vi "Main.vi"() -> ()   [LabVIEW 2024]
doc: "This small application is only a proof of concept. When we have parameters or user data inside an application that could be modified (by the user) at run time, it is important that those changes are 'memorized' when the application is shut down. The next time the application is started it should keep the last configuration made. This is what this application does.\n\nEvery time the user changes the FP data, the changes are saved in the .ini file. If the user closes the application, the FP data is already saved in the .ini configuration file. The next time it is turned on, the data will be loaded again.\n\nIf the user modifies any tag or sector name, or any key name (or its value) in the configuration file (and saves these changes) at run time, the Update button updates this information in the FP of the application, it is the data of the gray fields. This may not be useful in a real application."
uses:
  controls/UI Data.ctl
  controls/ring data.ctl
  support/Message Queue/Enqueue Message (Array).vi
  support/Message Queue/Enqueue Message (Single).vi
  dependencies/read-write config ini string data.vi
  <vilib>/Utility/config.llb/Read Key (String).vi
  <vilib>/Utility/config.llb/Write Key (String).vi
  <vilib>/Utility/error.llb/Error Cluster From Error Code.vi
  <vilib>/ErrorRing/Error Ring.xnode
  support/Message Queue/Message Queue.lvlib
  support/User Event - Stop/User Event - Stop.lvlib
  dependencies/read-write config ini.lvlib
  <vilib>/Utility/config.llb/NI_LVConfig.lvlib
panel:
  in  "Capacity":u16(ring) items=["9k", "12k", "18k", "24k"]
  in  "Type":u16(ring) items=["AB ROS", "INVERTER AG", "INVERTER SAMSUNG"]
  in  "Chassis":u16(ring) items=["MIDEA", "TCL"]
  in  "Sequence":u16(ring) items=["LOW", "LOW,MID", "LOW,HIGH", "LOW,TURBO", "LOW,MID,HIGH", "LOW,MID,TURBO", "LOW,HIGH,TURBO", "LOW,MID,HIGH,TURBO"]
  out "Display value":string
  in  "Exit":bool
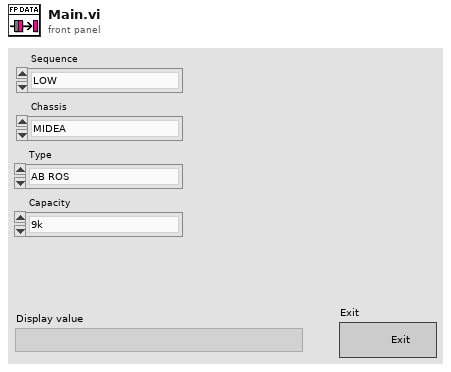
[diagram p1: front panel]
types:
  T1 = typedef "UI Data.ctl" = cluster{"Data Display Ref":refnum<vi>, "Exit Button Ref":refnum<vi>, "Ring Ref":refnum<vi>[], "types by chassis":T2, "ring opts":T2, "user ring data":T2, "actual chassis":string, "opt new type":cluster{"type":string, "key names":string[], "key values":string[]}}
  T2 = typedef "ring data.ctl" = cluster{"sectors":string[][], "key names":string[], "values":string[]}
  T3 = typedef "Message Queue.lvlib/All Message Queues.ctl" = cluster{"UI":refnum<queue>}
  T4 = cluster{"type":string, "key names":string[], "key values":string[]}
  T5 = typedef "NI_LVConfig.lvlib/Config Data RefNum.ctl" = refnum<k1>
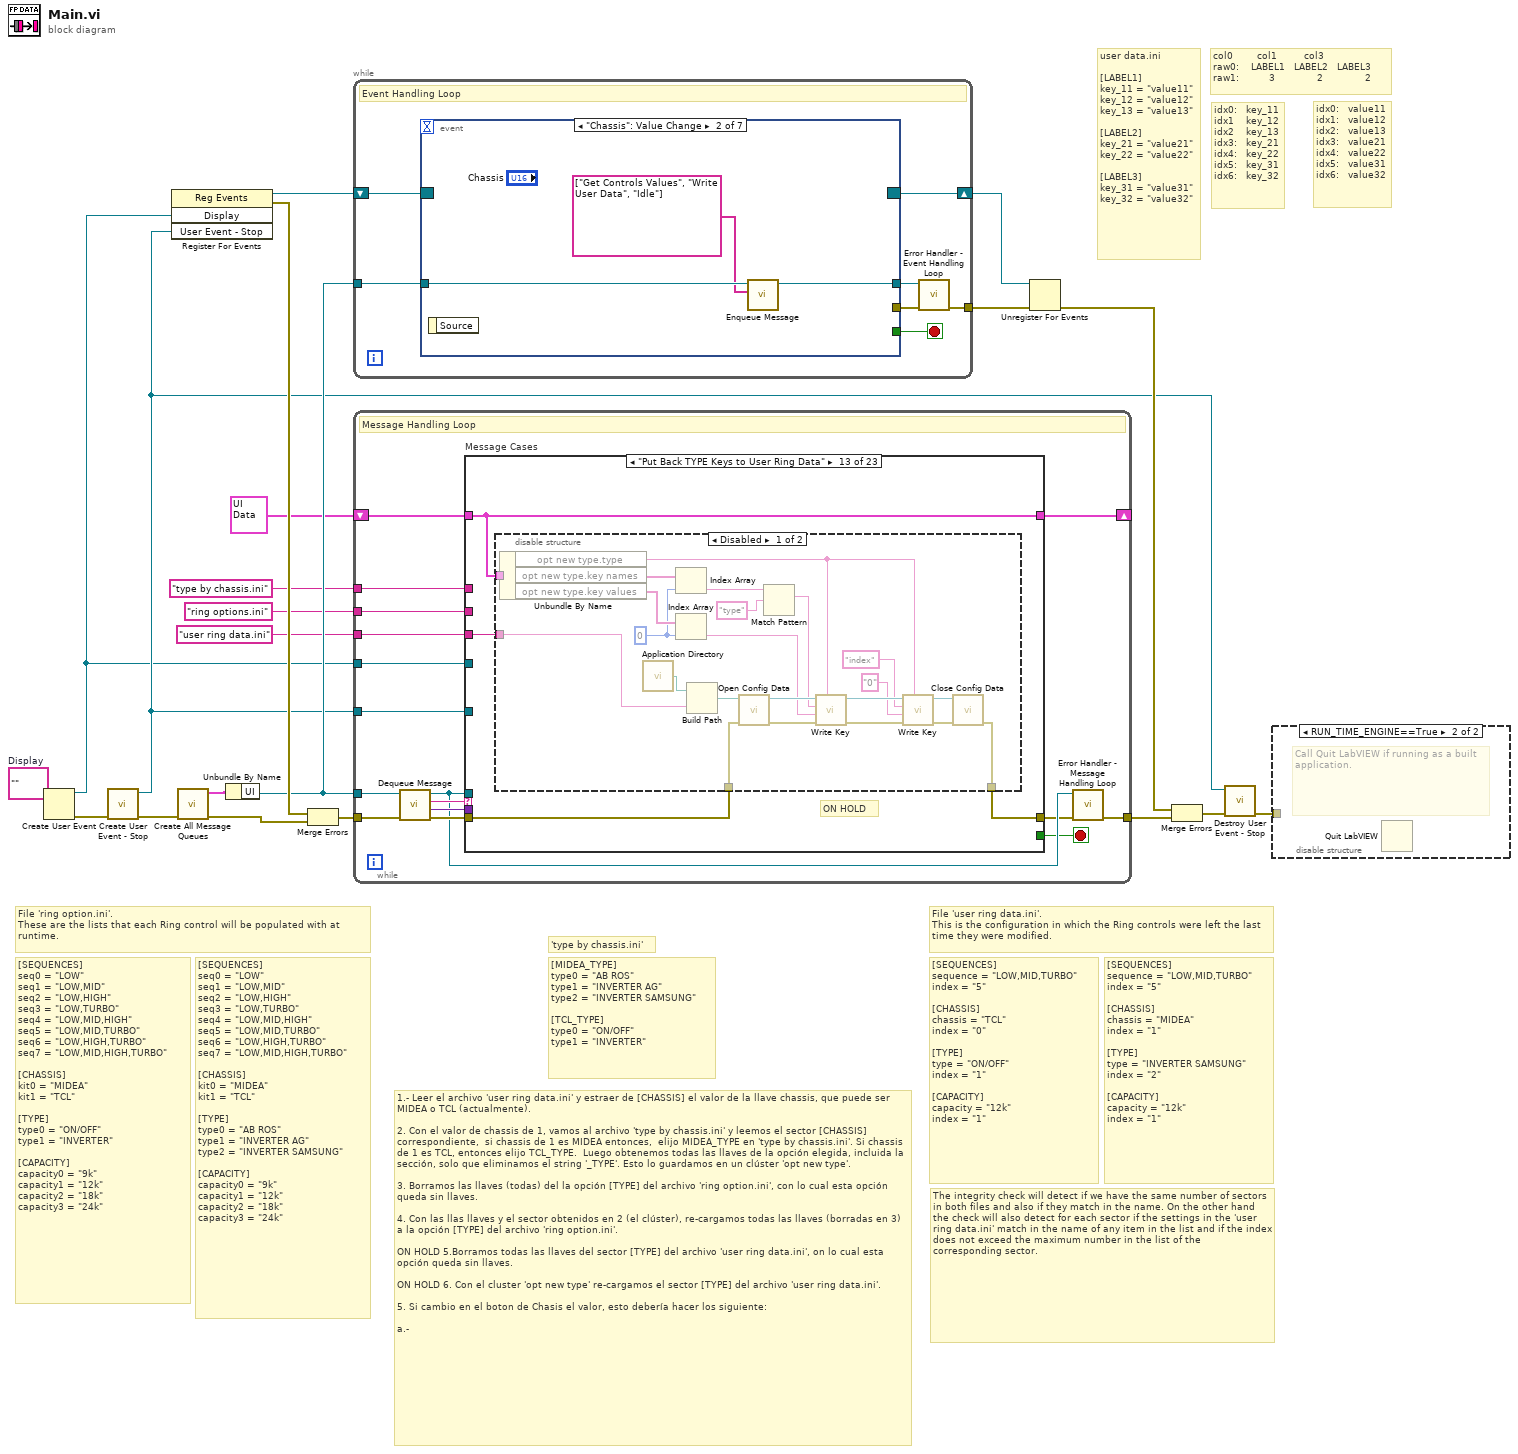
[diagram p0: block diagram]
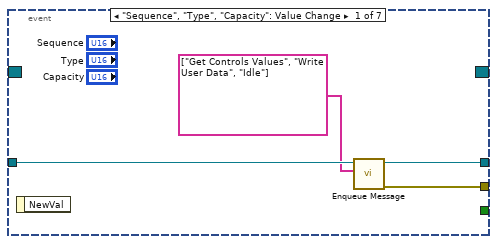
[diagram p3: hidden frame]
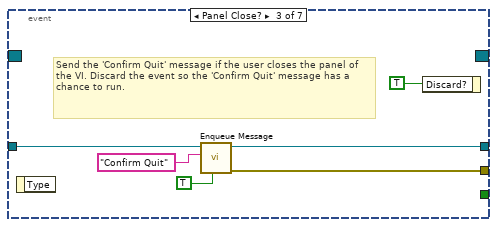
[diagram p4: hidden frame]
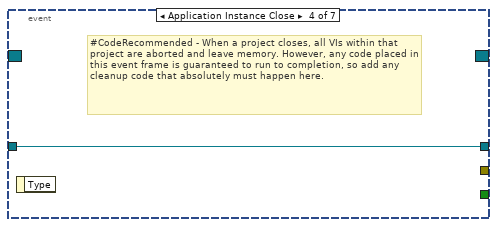
[diagram p5: hidden frame]
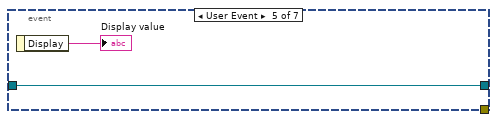
[diagram p6: hidden frame]
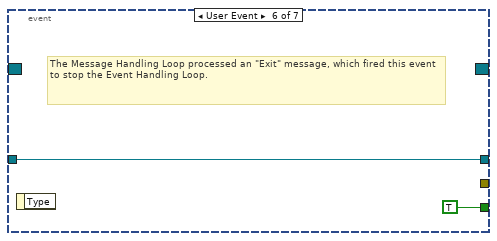
[diagram p7: hidden frame]
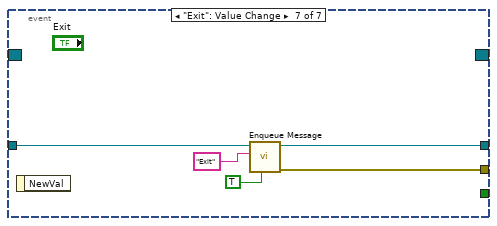
[diagram p8: hidden frame]
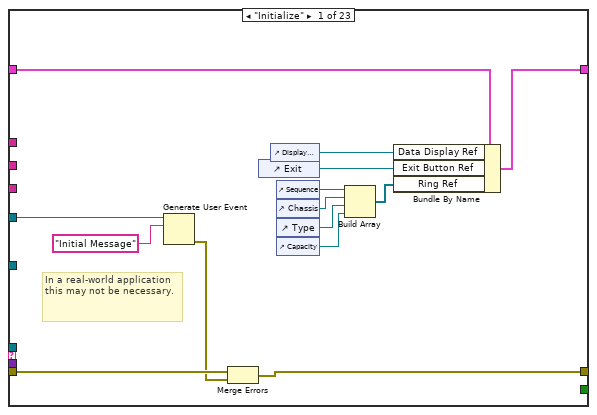
[diagram p9: hidden frame]
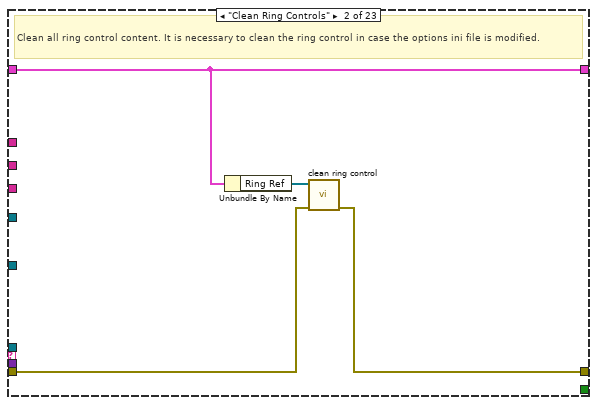
[diagram p10: hidden frame]
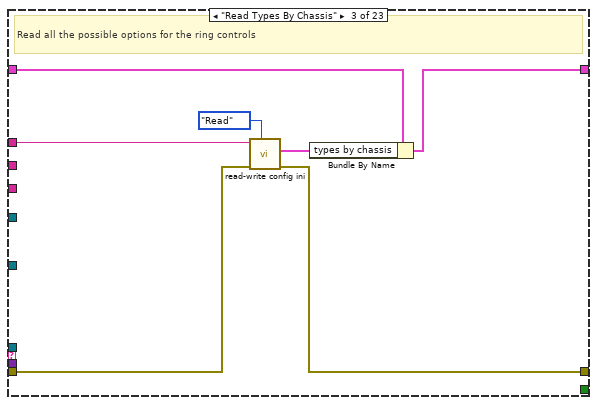
[diagram p11: hidden frame]
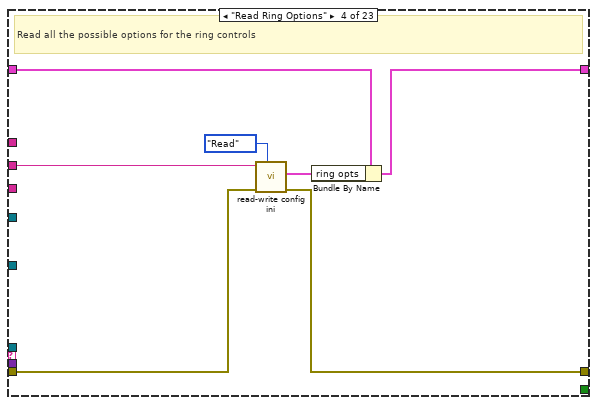
[diagram p12: hidden frame]
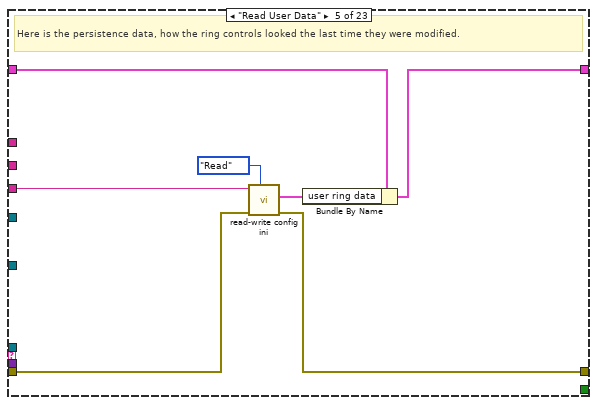
[diagram p13: hidden frame]
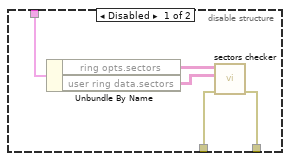
[diagram p15: hidden frame]
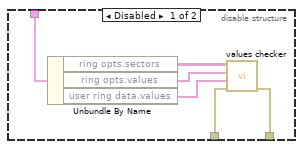
[diagram p17: hidden frame]
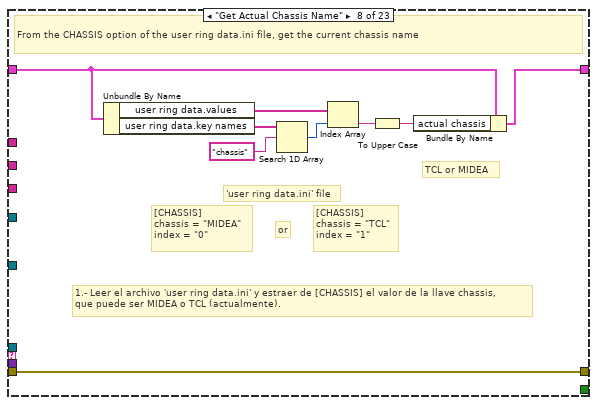
[diagram p18: hidden frame]
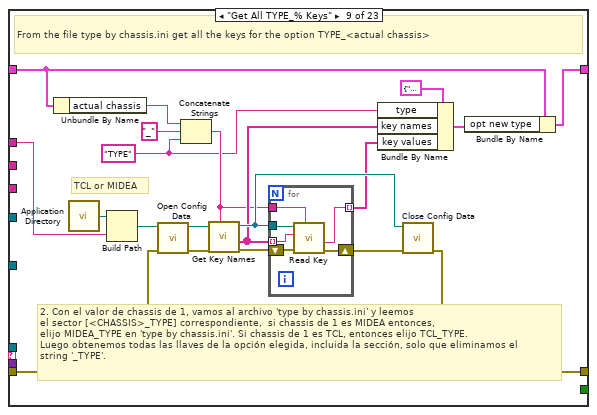
[diagram p19: hidden frame]
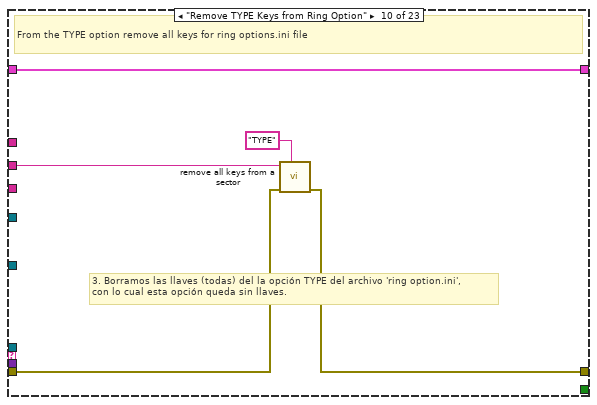
[diagram p20: hidden frame]
diagram:
  w6 = ""  # Display
  # "1.- Leer el archivo 'user ring data.ini' y estraer de [CHASSIS] el valor de la llave chassis, que puede ser MIDEA o TCL (actualmente).\n\n2. Con el valor de chassis de 1, vamos al archivo 'type by chassis.ini' y leemos el sector [CHASSIS] correspondiente,  si chassis de 1 es MIDEA entonces,  elijo MIDEA_TYPE en 'type by chassis.ini'. Si chassis de 1 es TCL, entonces elijo TCL_TYPE.  Luego obtenemos todas las llaves de la opción elegida, incluida la sección, solo que eliminamos el string '_TYPE'. Esto lo guardamos en un clúster 'opt new type'.\n\n3. Borramos las llaves (todas) del la opción [TYPE] del archivo 'ring option.ini', con lo cual esta opción queda sin llaves.\n\n4. Con las llas llaves y el sector obtenidos en 2 (el clúster), re-cargamos todas las llaves (borradas en 3) a la opción [TYPE] del archivo 'ring option.ini'.\n\nON HOLD 5.Borramos todas las llaves del sector [TYPE] del archivo 'user ring data.ini', on lo cual esta opción queda sin llaves.\n\nON HOLD 6. Con el cluster 'opt new type' re-cargamos el sector [TYPE] del archivo 'user ring data.ini'.\n\n5. Si cambio en el boton de Chasis el valor, esto debería hacer los siguiente:\n\na.-"
  # "[SEQUENCES]\nsequence = \"LOW,MID,TURBO\"\nindex = \"5\"\n\n[CHASSIS]\nchassis = \"MIDEA\"\nindex = \"1\"\n\n[TYPE]\ntype = \"INVERTER SAMSUNG\"\nindex = \"2\"\n\n[CAPACITY]\ncapacity = \"12k\"\nindex = \"1\""
  # "[SEQUENCES]\nseq0 = \"LOW\"\nseq1 = \"LOW,MID\"\nseq2 = \"LOW,HIGH\"\nseq3 = \"LOW,TURBO\"\nseq4 = \"LOW,MID,HIGH\"\nseq5 = \"LOW,MID,TURBO\"\nseq6 = \"LOW,HIGH,TURBO\"\nseq7 = \"LOW,MID,HIGH,TURBO\"\n\n[CHASSIS]\nkit0 = \"MIDEA\"\nkit1 = \"TCL\"\n\n[TYPE]\ntype0 = \"ON/OFF\"\ntype1 = \"INVERTER\"\n\n[CAPACITY]\ncapacity0 = \"9k\"\ncapacity1 = \"12k\"\ncapacity2 = \"18k\"\ncapacity3 = \"24k\""
  # "[MIDEA_TYPE]\ntype0 = \"AB ROS\"\ntype1 = \"INVERTER AG\"\ntype2 = \"INVERTER SAMSUNG\"\n\n[TCL_TYPE]\ntype0 = \"ON/OFF\"\ntype1 = \"INVERTER\""
  # "'type by chassis.ini'"
  # "The integrity check will detect if we have the same number of sectors in both files and also if they match in the name. On the other hand the check will also detect for each sector if the settings in the 'user ring data.ini' match in the name of any item in the list and if the index does not exceed the maximum number in the list of the corresponding sector."
  # "File 'user ring data.ini'.\nThis is the configuration in which the Ring controls were left the last time they were modified."
  # "[SEQUENCES]\nsequence = \"LOW,MID,TURBO\"\nindex = \"5\"\n\n[CHASSIS]\nchassis = \"TCL\"\nindex = \"0\"\n\n[TYPE]\ntype = \"ON/OFF\"\nindex = \"1\"\n\n[CAPACITY]\ncapacity = \"12k\"\nindex = \"1\""
  # "File 'ring option.ini'.\nThese are the lists that each Ring control will be populated with at runtime."
  # "[SEQUENCES]\nseq0 = \"LOW\"\nseq1 = \"LOW,MID\"\nseq2 = \"LOW,HIGH\"\nseq3 = \"LOW,TURBO\"\nseq4 = \"LOW,MID,HIGH\"\nseq5 = \"LOW,MID,TURBO\"\nseq6 = \"LOW,HIGH,TURBO\"\nseq7 = \"LOW,MID,HIGH,TURBO\"\n\n[CHASSIS]\nkit0 = \"MIDEA\"\nkit1 = \"TCL\"\n\n[TYPE]\ntype0 = \"AB ROS\"\ntype1 = \"INVERTER AG\"\ntype2 = \"INVERTER SAMSUNG\"\n\n[CAPACITY]\ncapacity0 = \"9k\"\ncapacity1 = \"12k\"\ncapacity2 = \"18k\"\ncapacity3 = \"24k\""
  # "user data.ini\n\n[LABEL1]\nkey_11 = \"value11\"\nkey_12 = \"value12\"\nkey_13 = \"value13\"\n\n[LABEL2]\nkey_21 = \"value21\"\nkey_22 = \"value22\"\n\n[LABEL3]\nkey_31 = \"value31\"\nkey_32 = \"value32\""
  # "idx0:   value11\nidx1:   value12\nidx2:   value13\nidx3:   value21\nidx4:   value22\nidx5:   value31\nidx6:   value32"
  # "idx0:   key_11\nidx1    key_12\nidx2    key_13\nidx3:   key_21\nidx4:   key_22\nidx5:   key_31\nidx6:   key_32"
  # "col0        col1         col3   \nraw0:    LABEL1   LABEL2   LABEL3\nraw1:          3              2              2"
  n1 = Create User Event(user event datatype=w6) -> (user event=w4:refnum<user-event>, error out=w7:errorcluster)  [unwired: 1 in]
  n2 = call "Create User Event - Stop.vi"("error in (no error)"=w7) -> ("error out"=w16:errorcluster, "User Event - Stop"=w5:refnum<user-event>)  [unwired: 9 in]
  n3 = register-events(w4, w5) -> (reference out=w9:refnum<event-registration>, error out=w21:errorcluster)  [unwired: 2 in]
  n4 = call "Create All Message Queues.vi"("error in (no error)"=w16) -> ("error out"=w20:errorcluster, "Message Queues out"=w19:T3)  [unwired: 9 in]
  n5 = Unbundle By Name(w19) -> ("UI"=w17:refnum<queue>)
  n6 = Merge Errors(w21, w20) -> (w8:errorcluster)
  n7 = while {
    tunnel: w17 -> [w28]
    shift-right: [w26] -> w13
    shift-left: w9 -> [w27]
    tunnel: [w22] -> w10
    stop <- w24 stop-if-true
    # "Event Handling Loop"
    n8 = event shown="[1] \"Chassis\": Value Change" {
      selector: w27 -> [_ _ _ _ _ _ _]
      dyn-events: [_ _ _ _ _ _ _] -> w26
      timeout: _ -> [_ _ _ _ _ _ _]
      tunnel: [_ _ _ _ _ TRUE ("Discard?") _] -> w24
      tunnel: w28 -> [w32 w35 w40 w42 w44 w46 w51]
      tunnel: [w30 _ w39 _ _ _ w50] -> w25
      tunnel: [w31 w34 w38 w42 w44 w46 w49] -> w23
      event "Sequence", "Type", "Capacity": Value Change {
        n9 = event-data() -> ()  [unwired: 1 in, 1 out]
        n10 = call-poly "Enqueue Message.vi"("Message Array"=string[] ["Get Controls Values", "Write User Data", "Idle"], "Message Queue"=w32) -> ("error out"=w30:errorcluster, "dup Message Queue"=w31:refnum<queue>)  [unwired: 8 in]
      }
      event "Chassis": Value Change {
        n11 = event-data() -> ()  [unwired: 1 in, 1 out]
        n12 = call-poly "Enqueue Message.vi"("Message Array"=string[] ["Get Controls Values", "Write User Data", "Idle"], "Message Queue"=w35) -> ("dup Message Queue"=w34:refnum<queue>)  [unwired: 8 in, 1 out]
      }
      event Panel Close? {
        # "Send the 'Confirm Quit' message if the user closes the panel of the VI. Discard the event so the 'Confirm Quit' message has a chance to run."
        n13 = event-data() -> ()  [unwired: 1 in, 1 out]
        n14 = call-poly "Enqueue Message.vi"("Priority Message? (F)"=TRUE, "Message"="Confirm Quit", "Message Queue"=w40) -> ("error out"=w39:errorcluster, "dup Message Queue"=w38:refnum<queue>)  [unwired: 7 in]
        n15 = event-data("Discard?"=TRUE) -> ()  [unwired: 1 in, 1 out]
      }
      event Application Instance Close {
        # "#CodeRecommended - When a project closes, all VIs within that project are aborted and leave memory. However, any code placed in this event frame is guaranteed to run to completion, so add any cleanup code that absolutely must happen here."
        n16 = event-data() -> ()  [unwired: 1 in, 1 out]
      }
      event User Event {
        n17 = event-data() -> ("Display"=→"Display value":string)  [unwired: 1 in]
      }
      event User Event {
        # "The Message Handling Loop processed an \"Exit\" message, which fired this event to stop the Event Handling Loop."
        n18 = event-data() -> ()  [unwired: 1 in, 1 out]
      }
      event "Exit": Value Change {
        n19 = event-data() -> ()  [unwired: 1 in, 1 out]
        n20 = call-poly "Enqueue Message.vi"("Priority Message? (F)"=TRUE, "Message"="Exit", "Message Queue"=w51) -> ("error out"=w50:errorcluster, "dup Message Queue"=w49:refnum<queue>)  [unwired: 7 in]
      }
    }
    n21 = call "Error Handler - Event Handling Loop.vi"("error in (no error)"=w25, "Message Queue"=w23) -> ("dup error in"=w22:errorcluster)  [unwired: 8 in, 1 out]
  }
  n22 = while {
    tunnel: w17 -> [w61]
    shift-right: [w56] -> _
    shift-left: T1 {"Data Display Ref"=refnum, "Exit Button Ref"=refnum, "Ring Ref"=[], "types by chassis"={"sectors"=[], "key names"=[], "values"=[]}, "ring opts"={"sectors"=[], "key names"=[], "values"=[]}, "user ring data"={"sectors"=[], "key names"=[], "values"=[]}, "actual chassis"="", "opt new type"={"type"="", "key names"=[], "key values"=[]}} ("Data Cluster") -> [w67]
    tunnel: w5 -> [w66]
    tunnel: w8 -> [w65]
    tunnel: [w59] -> w18
    tunnel: w4 -> [w57]
    tunnel: "user ring data.ini" -> [w55]
    tunnel: "ring options.ini" -> [w53]
    tunnel: "type by chassis.ini" -> [w52]
    stop <- w54 stop-if-true
    # "Message Handling Loop"
    n23 = call "Dequeue Message.vi"("error in (no error)"=w65, "Message Queue"=w61) -> ("error out"=w64:errorcluster, "Message Data"=w62:variant, "Message"=w63:string, "dup Message Queue"=w60:refnum<queue>)  [unwired: 6 in]
    n24 = case "Message Cases" shown="\"Put Back TYPE Keys to User Ring Data\"" w63 {
      selector: w63 -> [_ _ _ _ _ _ _ _ _ _ _ _ _ _ _ _ _ _ _ _ _ _ w281]
      tunnel: w60 -> [_ _ _ _ _ _ _ _ _ _ _ _ _ _ _ _ _ _ _ w259 _ w280 _]
      tunnel: w64 -> [w77 w83 w91 w97 w102 w108 w116 w132 w144 w162 w172 w183 w192 w220 w226 w232 w234 w244 w256 w263 w266 w273 _]
      tunnel: [w74 w82 w90 w96 w101 w107 w115 w132 w143 w161 w164 w182 w191 w219 w225 w231 w235 w248 w250 w261 w264 w276 w282] -> w58
      tunnel: w67 -> [w81 w85 w89 w95 w106 w109 w117 w127 w139 w163 w171 w185 w193 w218 w224 w230 w240 w249 w255 w262 w265 w279 w283]
      tunnel: [w80 w85 w87 w93 w105 w109 w117 w126 w137 w163 w171 w185 w193 w218 w224 w229 w240 w249 w255 w262 w265 w279 w283] -> w56
      tunnel: [_ _ _ _ _ _ _ _ _ _ _ _ _ _ _ _ _ _ _ _ _ TRUE _] -> w54
      tunnel: w62 -> [_ _ _ _ _ _ _ _ _ _ _ _ _ _ _ _ _ w245 w254 _ _ w270 _]
      tunnel: w66 -> [_ _ _ _ _ _ _ _ _ _ _ _ _ _ _ _ _ _ _ _ _ w275 _]
      tunnel: w57 -> [w76 _ _ _ _ _ _ _ _ _ _ _ _ _ _ _ _ w247 _ _ _ w268 _]
      tunnel: w55 -> [_ _ _ _ w104 _ _ _ _ _ _ w184 w190 _ _ _ w239 _ _ _ _ _ _]
      tunnel: w53 -> [_ _ _ w99 _ _ _ _ _ w159 w173 _ _ _ _ _ _ _ _ _ _ _ _]
      tunnel: w52 -> [_ _ w86 _ _ _ _ _ w149 _ _ _ _ _ _ _ _ _ _ _ _ _ _]
      frame "Initialize" {
        # "In a real-world application this may not be necessary."
        n25 = Generate User Event(user event=w76, event data cluster="Initial Message" ("Initial Message")) -> (error out=w73:errorcluster)  [unwired: 2 in, 1 out]
        n26 = Merge Errors(w77, w73) -> (w74:errorcluster)
        n27 = control-ref of="Exit"() -> (w78:refnum<vi>)
        n28 = control-ref of="Display value"() -> (w79:refnum<vi>)
        n29 = control-ref of="Sequence"() -> (w72:refnum<vi>)
        n30 = control-ref of="Chassis"() -> (w71:refnum<vi>)
        n31 = control-ref of="Type"() -> (w70:refnum<vi>)
        n32 = control-ref of="Capacity"() -> (w68:refnum<vi>)
        n33 = Build Array(w72, w71, w70, w68) -> (w69:refnum<vi>[])
        n34 = Bundle By Name(cluster=w81, "Data Display Ref"=w79, "Exit Button Ref"=w78, "Ring Ref"=w69) -> (w80:T1)
      }
      frame "Clean Ring Controls" {
        # "Clean all ring control content. It is necessary to clean the ring control in case the options ini file is modified."
        n35 = Unbundle By Name(w85) -> ("Ring Ref"=w84:refnum<vi>[])
        n36 = call "clean ring control.vi"("error in (no error)"=w83, "Ring Ref"=w84) -> ("error out"=w82:errorcluster)  [unwired: 9 in]
      }
      frame "Read Types By Chassis" {
        # "Read all the possible options for the ring controls"
        n37 = call-poly "read-write config ini.vi"("Function"=enum16{"Read", "Write"}."Read", "error in (no error)"=w91, "file name"=w86) -> ("error out"=w90:errorcluster, "user data out"=w88:T2)  [unwired: 7 in]
        n38 = Bundle By Name(cluster=w89, "types by chassis"=w88) -> (w87:T1)
      }
      frame "Read Ring Options" {
        # "Read all the possible options for the ring controls"
        n39 = call-poly "read-write config ini.vi"("Function"=enum16{"Read", "Write"}."Read", "error in (no error)"=w97, "file name"=w99) -> ("error out"=w96:errorcluster, "user data out"=w94:T2)  [unwired: 7 in]
        n40 = Bundle By Name(cluster=w95, "ring opts"=w94) -> (w93:T1)
      }
      frame "Read User Data" {
        # "Here is the persistence data, how the ring controls looked the last time they were modified."
        n41 = call-poly "read-write config ini.vi"("Function"=enum16{"Read", "Write"}."Read", "error in (no error)"=w102, "file name"=w104) -> ("error out"=w101:errorcluster, "user data out"=w100:T2)  [unwired: 7 in]
        n42 = Bundle By Name(cluster=w106, "user ring data"=w100) -> (w105:T1)
      }
      frame "Check for Sectors" {
        # "Verifying configuration files integrity"
        n43 = disable-structure shown="Enabled" {
          disable-tunnel: w109 -> [w112 _]
          disable-tunnel: w108 -> [w111 _]
          disable-tunnel: [w110 _] -> w107
          frame Disabled {
            n44 = Unbundle By Name(w112) -> ("ring opts.sectors"=w114:string[][], "user ring data.sectors"=w113:string[][])
            n45 = call "sectors checker.vi"("error in (no error)"=w111, "array2"=w113, "array1"=w114) -> ("error out"=w110:errorcluster)  [unwired: 8 in]
          }
          frame Enabled {
          }
        }
      }
      frame "Check For Values" {
        # "Verifying configuration files integrity"
        n46 = disable-structure shown="Enabled" {
          disable-tunnel: w117 -> [w120 _]
          disable-tunnel: w116 -> [w119 _]
          disable-tunnel: [w118 _] -> w115
          frame Disabled {
            n47 = Unbundle By Name(w120) -> ("ring opts.sectors"=w123:string[][], "ring opts.values"=w122:string[], "user ring data.values"=w121:string[])
            n48 = call "values checker.vi"("error in (no error)"=w119, "values"=w121, "values 2"=w122, "sectors"=w123) -> ("error out"=w118:errorcluster)  [unwired: 7 in]
          }
          frame Enabled {
          }
        }
      }
      frame "Get Actual Chassis Name" {
        # "1.- Leer el archivo 'user ring data.ini' y estraer de [CHASSIS] el valor de la llave chassis, \nque puede ser MIDEA o TCL (actualmente)."
        # "TCL or MIDEA"
        # "'user ring data.ini' file"
        # "or"
        # "[CHASSIS]\nchassis = \"MIDEA\"\nindex = \"0\""
        # "[CHASSIS]\nchassis = \"TCL\"\nindex = \"1\""
        # "From the CHASSIS option of the user ring data.ini file, get the current chassis name"
        n49 = Unbundle By Name(w127) -> ("user ring data.values"=w129:string[], "user ring data.key names"=w131:string[])
        n50 = Search 1D Array(1D array=w131, element="chassis") -> (index of element=w128:i32)  [unwired: 1 in]
        n51 = Index Array(array=w129, index=w128) -> (element=w125:string)
        n52 = To Upper Case(1:w125) -> (0:w124:string)
        n53 = Bundle By Name(cluster=w127, "actual chassis"=w124) -> (w126:T1)
      }
      frame "Get All TYPE_% Keys" {
        w133 = "TYPE"
        # "2. Con el valor de chassis de 1, vamos al archivo 'type by chassis.ini' y leemos\nel sector [<CHASSIS>_TYPE] correspondiente,  si chassis de 1 es MIDEA entonces,  \nelijo MIDEA_TYPE en 'type by chassis.ini'. Si chassis de 1 es TCL, entonces elijo TCL_TYPE. \nLuego obtenemos todas las llaves de la opción elegida, incluida la sección, solo que eliminamos el \nstring '_TYPE'."
        # "TCL or MIDEA"
        # "From the file type by chassis.ini get all the keys for the option TYPE_<actual chassis>"
        n54 = Unbundle By Name(w139) -> ("actual chassis"=w134:string)
        n55 = call <vilib>:"Application Directory.vi"() -> ("Application Directory"=w151:path)
        n56 = Build Path(base path=w151, name or relative path=w149) -> (appended path=w150:path)
        n57 = call <vilib>:"Open Config Data.vi"("error in (no error)"=w144, "configuration file path"=w150) -> ("error out"=w148:errorcluster, "refnum"=w147:T5)  [unwired: 7 in, 1 out]
        n58 = Concatenate Strings(w134, "_", w133) -> (w136:string)
        n59 = call <vilib>:"Get Key Names.vi"("section"=w136, "error in (no error)"=w148, "refnum"=w147) -> ("error out"=w146:errorcluster, "key names"=w141:string[], "refnum out"=w152:T5)  [unwired: 5 in, 1 out]
        n60 = for {
          tunnel: w141 -> [w157] mode=indexing
          tunnel: w152 -> [w158]
          tunnel: w136 -> [w156]
          tunnel: [w155] -> w140 mode=indexing
          shift-right: [w153] -> w145
          shift-left: w146 -> [w154]
          n61 = call-poly <vilib>:"Read Key.vi"("section"=w156, "error in (no error)"=w154, "key"=w157, "refnum"=w158) -> ("error out"=w153:errorcluster, "value"=w155:string)  [unwired: 4 in, 2 out]
        }
        n62 = Bundle By Name(cluster=T4 {"type"="", "key names"=[], "key values"=[]}, "type"=w133, "key names"=w141, "key values"=w140) -> (w138:T4)
        n63 = call <vilib>:"Close Config Data.vi"("error in (no error)"=w145, "refnum"=w152) -> ("error out"=w143:errorcluster)  [unwired: 8 in, 1 out]
        n64 = Bundle By Name(cluster=w139, "opt new type"=w138) -> (w137:T1)
      }
      frame "Remove TYPE Keys from Ring Option" {
        # "3. Borramos las llaves (todas) del la opción TYPE del archivo 'ring option.ini', \ncon lo cual esta opción queda sin llaves."
        # "From the TYPE option remove all keys for ring options.ini file"
        n65 = call "remove all keys from a sector.vi"("sector"="TYPE", "error in (no error)"=w162, "file name"=w159) -> ("error out"=w161:errorcluster)  [unwired: 8 in]
      }
      frame "Put Back TYPE Keys to Ring Option" {
        # "4. Con las llas llaves y el sector obtenidos en 2, re-cargar todas las llaves (borradas en 3)\na la opción TYPE del archivo 'ring option.ini'."
        n66 = Unbundle By Name(w171) -> ("opt new type.type"=w169:string, "opt new type.key names"=w167:string[], "opt new type.key values"=w168:string[])
        n67 = call <vilib>:"Application Directory.vi"() -> ("Application Directory"=w174:path)
        n68 = Build Path(base path=w174, name or relative path=w173) -> (appended path=w175:path)
        n69 = call <vilib>:"Open Config Data.vi"("error in (no error)"=w172, "configuration file path"=w175) -> ("error out"=w170:errorcluster, "refnum"=w165:T5)  [unwired: 7 in, 1 out]
        n70 = for {
          tunnel: w165 -> [w180]
          tunnel: w169 -> [w179]
          shift-right: [w178] -> w166
          shift-left: w170 -> [w181]
          tunnel: w168 -> [w177] mode=indexing
          tunnel: w167 -> [w176] mode=indexing
          n71 = call-poly <vilib>:"Write Key.vi"("section"=w179, "error in (no error)"=w181, "value"=w177, "key"=w176, "refnum"=w180) -> ("error out"=w178:errorcluster)  [unwired: 4 in, 2 out]
        }
        n72 = call <vilib>:"Close Config Data.vi"("error in (no error)"=w166, "refnum"=w165) -> ("error out"=w164:errorcluster)  [unwired: 8 in, 1 out]
      }
      frame "Remove TYPE Keys from User Ring Data" {
        # "ON HOLD"
        # "5.Borramos todas las llaves del sector [TYPE] del archivo 'user ring data.ini', on lo cual esta opción queda sin llaves."
        n73 = disable-structure shown="Disabled" {
          disable-tunnel: w184 -> [w188 _]
          disable-tunnel: w183 -> [w187 _]
          disable-tunnel: [w186 _] -> w182
          frame Disabled {
            n74 = call "remove all keys from a sector.vi"("sector"="TYPE", "error in (no error)"=w187, "file name"=w188) -> ("error out"=w186:errorcluster)  [unwired: 8 in]
          }
          frame Enabled {
          }
        }
      }
      frame "Put Back TYPE Keys to User Ring Data" {
        # "ON HOLD"
        n75 = disable-structure shown="Disabled" {
          disable-tunnel: w193 -> [w215 _]
          disable-tunnel: w192 -> [w212 _]
          disable-tunnel: [w205 _] -> w191
          disable-tunnel: w190 -> [w197 _]
          frame Disabled {
            w207 = 0 ("index")
            n76 = Unbundle By Name(w215) -> ("opt new type.type"=w202:string, "opt new type.key names"=w209:string[], "opt new type.key values"=w208:string[])
            n77 = call <vilib>:"Application Directory.vi"() -> ("Application Directory"=w214:path)
            n78 = Index Array(array=w209, index=w207) -> (element=w196:string)
            n79 = Index Array(array=w208, index=w207) -> (element=w206:string)
            n80 = Build Path(base path=w214, name or relative path=w197) -> (appended path=w213:path)
            n81 = call <vilib>:"Open Config Data.vi"("error in (no error)"=w212, "configuration file path"=w213) -> ("error out"=w211:errorcluster, "refnum"=w210:T5)  [unwired: 7 in, 1 out]
            n82 = Match Pattern(string=w196, regular expression="type") -> (match substring=w194:string)  [unwired: 1 in, 3 out]
            n83 = call-poly <vilib>:"Write Key.vi"("section"=w202, "error in (no error)"=w211, "value"=w206, "key"=w194, "refnum"=w210) -> ("error out"=w204:errorcluster, "refnum out"=w201:T5)  [unwired: 4 in, 1 out]
            n84 = call-poly <vilib>:"Write Key.vi"("section"=w202, "error in (no error)"=w204, "value"="0", "key"="index", "refnum"=w201) -> ("error out"=w203:errorcluster, "refnum out"=w200:T5)  [unwired: 4 in, 1 out]
            n85 = call <vilib>:"Close Config Data.vi"("error in (no error)"=w203, "refnum"=w200) -> ("error out"=w205:errorcluster)  [unwired: 8 in, 1 out]
          }
          frame Enabled {
          }
        }
      }
      frame "Fill Ring Controls with Options" {
        # "WARNING: This process is position dependent. That is, how the ring control references are placed into the Ring Ref array."
        # "Set all options on the ring controls."
        n86 = Unbundle By Name(w218) -> ("Ring Ref"=w217:refnum<vi>[], "ring opts"=w216:T2)
        n87 = call "fill ring control with options.vi"("error in (no error)"=w220, "ring options"=w216, "Ring Ref"=w217) -> ("error out"=w219:errorcluster)  [unwired: 8 in]
      }
      frame "Set Controls Values" {
        # "WARNING: This process is position dependent. That is, how the ring control references are placed into the Ring Ref array."
        # "This diagram is used to update the persistance data in the FP controls after reading the .ini file."
        n88 = Unbundle By Name(w224) -> ("Ring Ref"=w223:refnum<vi>[], "user ring data"=w222:T2)
        n89 = call "set and get ring values.vi"("function"=enum16{"Set", "Get"}."Set", "error in (no error)"=w226, "user options"=w222, "Ring Ref"=w223) -> ("error out"=w225:errorcluster)  [unwired: 6 in, 1 out]
      }
      frame "Get Controls Values" {
        # "WARNING: This process is position dependent. That is, how the ring control references are placed into the Ring Ref array."
        # "Here we read the current positions of the ring controls, and store them in the Data Highway."
        n90 = Unbundle By Name(w230) -> ("Ring Ref"=w233:refnum<vi>[])
        n91 = call "set and get ring values.vi"("function"=enum16{"Set", "Get"}."Get", "error in (no error)"=w232, "Ring Ref"=w233) -> ("error out"=w231:errorcluster, "values & indexes"=w228:string[])  [unwired: 7 in]
        n92 = Bundle By Name(cluster=w230, "user ring data.values"=w228) -> (w229:T1)
      }
      frame "Write User Data" {
        # "In this diagram all persistance data is written to the .ini configuration file."
        n93 = Unbundle By Name(w240) -> ("user ring data"=w238:T2)
        n94 = call-poly "read-write config ini.vi"("Function"=enum16{"Read", "Write"}."Write", "error in (no error)"=w234, "user data in"=w238, "file name"=w239) -> ("error out"=w236:errorcluster)  [unwired: 6 in, 1 out]
        n95 = Merge Errors(w236) -> (w235:errorcluster)
      }
      frame "Update Display" {
        # "In a real-world application this may not be necessary."
        # "Update Display - Convert the message data to a string to display in the Data Display indicator."
        n96 = Variant To Data(error in=w244, type="", Variant=w245) -> (data=w241:string, error out=w243:errorcluster)
        n97 = Generate User Event(user event=w247, event data cluster=w241) -> (error out=w246:errorcluster)  [unwired: 2 in, 1 out]
        n98 = Merge Errors(w243, w246) -> (w248:errorcluster)
      }
      frame "Error" {
        # "#CodeRecommended - If you ever change the name of this \"Error\" message, you'll need to update the name in the Check Loop Error.vi as well."
        # "#CodeRecommended - Consider creating a system for logging errors in some way. These errors are for notification purposes only. Handling of specific errors should be performed in the message frames that generated the error."
        # "Error - Display an error dialog. This message is sent by the \"Error Handler\" VIs at the end of other loops in this application."
        n99 = Variant To Data(error in=w256, type=errorcluster {"status"=FALSE, "code"=0, "source"=""} ("error constant"), Variant=w254) -> (data=w252:errorcluster, error out=w251:errorcluster)
        n100 = call <vilib>:"Simple Error Handler.vi"("error in (no error)"=w252) -> ()  [unwired: 4 in, 5 out]
        n101 = Merge Errors(w251) -> (w250:errorcluster)
      }
      frame "Confirm Quit" {
        # "#CodeNeeded - If you want to provide an \"Are you sure\" dialog (or some other notification) before the application exits, place that code here. This message is typically sent from a Panel Close? event."
        # "Confirm Quit - Message that can confirm whether or not the user wants to exit the application."
        n102 = call-poly "Enqueue Message.vi"("Priority Message? (F)"=TRUE, "error in (no error)"=w263, "Message"="Exit", "Message Queue"=w259) -> ("error out"=w260:errorcluster)  [unwired: 6 in, 1 out]
        n103 = Merge Errors(w260) -> (w261:errorcluster)
      }
      frame "Idle" {
        # "Idle diagram"
        n104 = Merge Errors(w266) -> (w264:errorcluster)
      }
      frame "Exit" {
        # "In a real-world application this may not be necessary."
        # "Release the message queue reference"
        # "#CodeNeeded - Add any required cleanup code here. Note that if 'Exit' was called as a result of an error, an error dialog will be displayed. Add any custom error handling for an 'Exit' condition here as well."
        # "Exit - Exit the application."
        n105 = Variant To Data(type=errorcluster {"status"=FALSE, "code"=0, "source"=""} ("error constant"), Variant=w270) -> (data=w271:errorcluster)  [unwired: 1 in, 1 out]
        n106 = call <vilib>:"Simple Error Handler.vi"("error in (no error)"=w271) -> ()  [unwired: 4 in, 5 out]
        n107 = Generate User Event(user event=w268, event data cluster="\"Exit\" button pressed" ("Initial Message")) -> (error out=w267:errorcluster)  [unwired: 2 in, 1 out]
        n108 = call "Fire User Event - Stop.vi"("User Event - Stop"=w275) -> ("error out"=w274:errorcluster)  [unwired: 10 in]
        n109 = Release Queue(queue=w280, error in (no error)=w273) -> (error out=w277:errorcluster)  [unwired: 1 in, 2 out]
        n110 = Merge Errors(w267, w274, w277) -> (w276:errorcluster)
      }
      frame Default {
        # "'Default' case only runs if there is a message that isn't defined in any of the other cases.\nOutput a programming error."
        n111 = xnode "Error Ring"("parameter 0"=w281) -> ("error out"=w282:errorcluster)
      }
    }
    n112 = call "Error Handler - Message Handling Loop.vi"("error in (no error)"=w58, "Message Queue"=w60) -> ("dup error in"=w59:errorcluster)  [unwired: 8 in, 1 out]
  }
  n113 = Unregister For Events(event registration refnum=w13, error in=w10) -> (error out=w14:errorcluster)
  n114 = Merge Errors(w14, w18) -> (w15:errorcluster)
  n115 = call "Destroy User Event - Stop.vi"("error in (no error)"=w15, "User Event - Stop"=w5) -> ("error out"=w11:errorcluster)  [unwired: 9 in]
  n116 = disable-structure shown="RUN_TIME_ENGINE==True" {
    disable-tunnel: w11 -> [_ _]
    frame condition #0 (active) {
    }
    frame condition #1 {
      # "Call Quit LabVIEW if running as a built application."
      n117 = Quit LabVIEW() -> ()  [unwired: 1 in]
    }
  }
